vi "启动条件判断.vi"(7 "时间源":T1, 8 "仪器状态":bool, 9 "启动次数":i32, 10 "间隔计时":i32, 11 "周期设置输出":T6 {"定点周期"."启动命令 24" items=["", "水样测试", "标样核查", "零点核查", "跨度核查", "空白测试", "平行样测试", "加标回收", "空白校准", "标样校准"]; "定点周期"."启动命令 23" items=["", "水样测试", "标样核查", "零点核查", "跨度核查", "空白测试", "平行样测试", "加标回收", "空白校准", "标样校准"]; "定点周期"."启动命令 22" items=["", "水样测试", "标样核查", "零点核查", "跨度核查", "空白测试", "平行样测试", "加标回收", "空白校准", "标样校准"]; "定点周期"."启动命令 21" items=["", "水样测试", "标样核查", "零点核查", "跨度核查", "空白测试", "平行样测试", "加标回收", "空白校准", "标样校准"]; "定点周期"."启动命令 20" items=["", "水样测试", "标样核查", "零点核查", "跨度核查", "空白测试", "平行样测试", "加标回收", "空白校准", "标样校准"]; "定点周期"."启动命令 19" items=["", "水样测试", "标样核查", "零点核查", "跨度核查", "空白测试", "平行样测试", "加标回收", "空白校准", "标样校准"]; "定点周期"."启动命令 18" items=["", "水样测试", "标样核查", "零点核查", "跨度核查", "空白测试", "平行样测试", "加标回收", "空白校准", "标样校准"]; "定点周期"."启动命令 17" items=["", "水样测试", "标样核查", "零点核查", "跨度核查", "空白测试", "平行样测试", "加标回收", "空白校准", "标样校准"]; "定点周期"."启动命令 16" items=["", "水样测试", "标样核查", "零点核查", "跨度核查", "空白测试", "平行样测试", "加标回收", "空白校准", "标样校准"]; "定点周期"."启动命令 15" items=["", "水样测试", "标样核查", "零点核查", "跨度核查", "空白测试", "平行样测试", "加标回收", "空白校准", "标样校准"]; "定点周期"."启动命令 14" items=["", "水样测试", "标样核查", "零点核查", "跨度核查", "空白测试", "平行样测试", "加标回收", "空白校准", "标样校准"]; "定点周期"."启动命令 13" items=["", "水样测试", "标样核查", "零点核查", "跨度核查", "空白测试", "平行样测试", "加标回收", "空白校准", "标样校准"]; "定点周期"."启动命令 12" items=["", "水样测试", "标样核查", "零点核查", "跨度核查", "空白测试", "平行样测试", "加标回收", "空白校准", "标样校准"]; "定点周期"."启动命令 11" items=["", "水样测试", "标样核查", "零点核查", "跨度核查", "空白测试", "平行样测试", "加标回收", "空白校准", "标样校准"]; "定点周期"."启动命令 10" items=["", "水样测试", "标样核查", "零点核查", "跨度核查", "空白测试", "平行样测试", "加标回收", "空白校准", "标样校准"]; "定点周期"."启动命令 9" items=["", "水样测试", "标样核查", "零点核查", "跨度核查", "空白测试", "平行样测试", "加标回收", "空白校准", "标样校准"]; "定点周期"."启动命令 8" items=["", "水样测试", "标样核查", "零点核查", "跨度核查", "空白测试", "平行样测试", "加标回收", "空白校准", "标样校准"]; "定点周期"."启动命令 7" items=["", "水样测试", "标样核查", "零点核查", "跨度核查", "空白测试", "平行样测试", "加标回收", "空白校准", "标样校准"]; "定点周期"."启动命令 6" items=["", "水样测试", "标样核查", "零点核查", "跨度核查", "空白测试", "平行样测试", "加标回收", "空白校准", "标样校准"]; "定点周期"."启动命令 5" items=["", "水样测试", "标样核查", "零点核查", "跨度核查", "空白测试", "平行样测试", "加标回收", "空白校准", "标样校准"]; "定点周期"."启动命令 4" items=["", "水样测试", "标样核查", "零点核查", "跨度核查", "空白测试", "平行样测试", "加标回收", "空白校准", "标样校准"]; "定点周期"."启动命令 3" items=["", "水样测试", "标样核查", "零点核查", "跨度核查", "空白测试", "平行样测试", "加标回收", "空白校准", "标样校准"]; "定点周期"."启动命令 2" items=["", "水样测试", "标样核查", "零点核查", "跨度核查", "空白测试", "平行样测试", "加标回收", "空白校准", "标样校准"]; "定点周期"."启动命令" items=["", "水样测试", "标样核查", "零点核查", "跨度核查", "空白测试", "平行样测试", "加标回收", "空白校准", "标样校准"]; "间隔设置"."启动命令" items=["", "水样测试", "标样核查", "零点核查", "跨度核查", "空白测试", "平行样测试", "加标回收", "空白校准", "标样校准"]}) -> (2 "重新配置":bool, 3 "Data":T7 caption="数据")   [LabVIEW 2016, in "定时设置.xctl"]
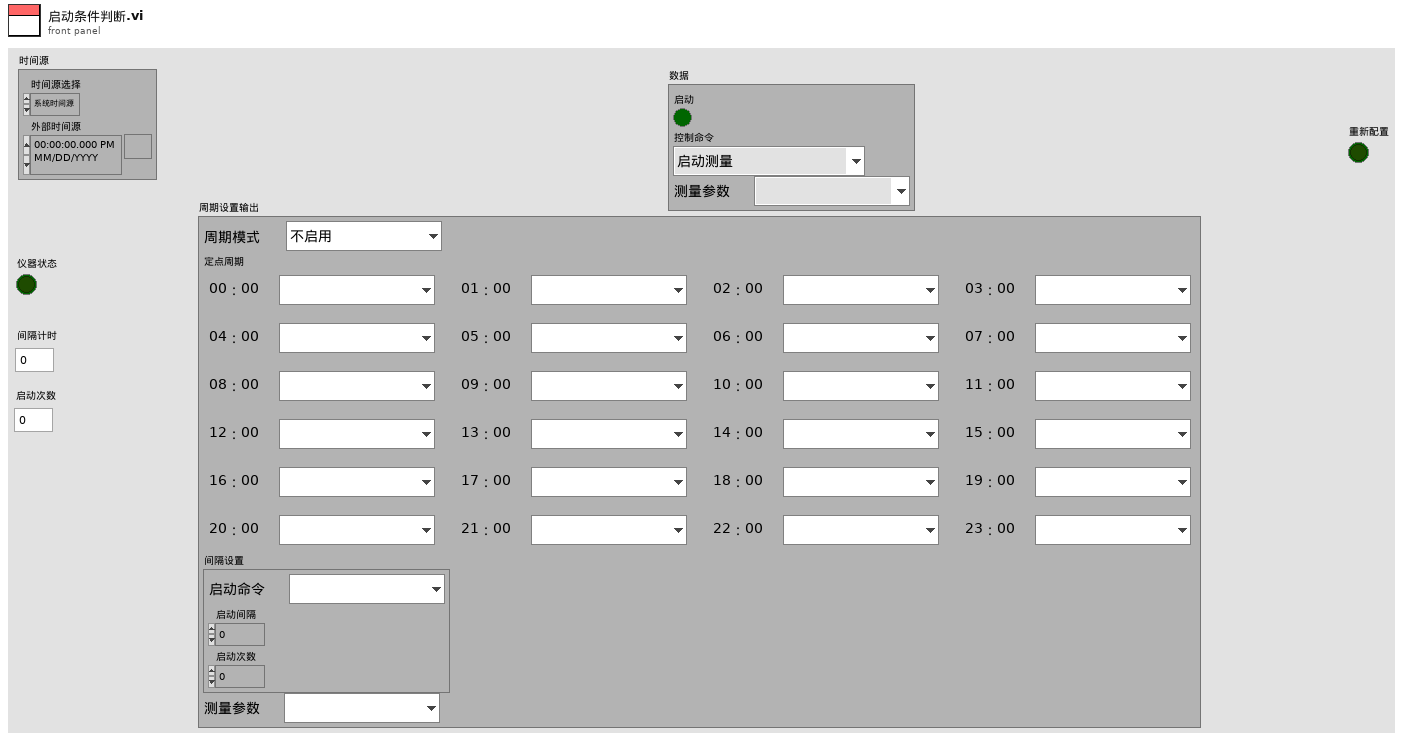
[diagram p1: front panel]
types:
  T1 = cluster{"时间源选择":enum16{"系统时间源", "仪器时间源"}, "外部时间源":timestamp}
  T2 = typedef "定时设置.xctl/周期模式设置.ctl" = enum16{"不启用", "定点模式", "间隔模式"}
  T3 = typedef "定时设置.xctl/定点周期设置.ctl" = cluster{"启动命令":T4, "启动命令 2":T4, "启动命令 3":T4, "启动命令 4":T4, "启动命令 5":T4, "启动命令 6":T4, "启动命令 7":T4, "启动命令 8":T4, "启动命令 9":T4, "启动命令 10":T4, "启动命令 11":T4, "启动命令 12":T4, "启动命令 13":T4, "启动命令 14":T4, "启动命令 15":T4, "启动命令 16":T4, "启动命令 17":T4, "启动命令 18":T4, "启动命令 19":T4, "启动命令 20":T4, "启动命令 21":T4, "启动命令 22":T4, "启动命令 23":T4, "启动命令 24":T4}
  T4 = typedef "定时设置.xctl/启动命令选择.ctl" = u16
  T5 = typedef "定时设置.xctl/测量参数.ctl" = u16
  T6 = cluster{"周期模式":T2, "定点周期":T3, "间隔设置":cluster{"启动命令":T4, "启动间隔":dbl, "启动次数":i32}, "测量参数":T5}
  T7 = typedef "定时设置.xctl/数据.ctl" = cluster{"启动":bool, "控制命令":T8, "测量参数":T5}
  T8 = typedef "定时设置.xctl/国标控制命令.ctl" = enum16{"启动测量", "标样核查", "零点核查", "跨度核查", "空白测试", "平行样测试", "加标回收", "空白校准", "标样校准", "初始化（清洗）", "停止测试", "仪器重启", "校时", "模式设置", "测量间隔设置"}
  T9 = typedef "LVDateTimeRec.ctl" = cluster{"秒数的小数部分":dbl, "秒":i32, "分":i32, "时":i32, "日":i32, "月":i32, "年":i32, "天数（周）":i32, "天数（年）":i32, "DST":i32}
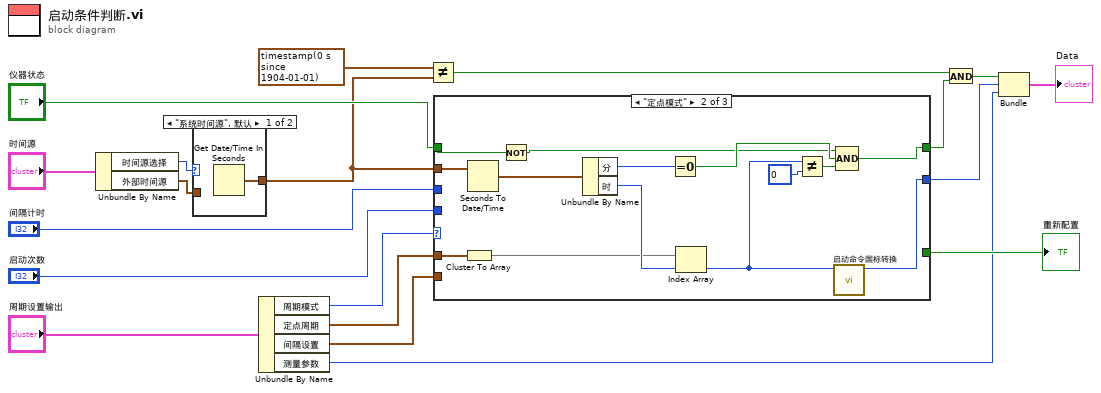
[diagram p0: block diagram]
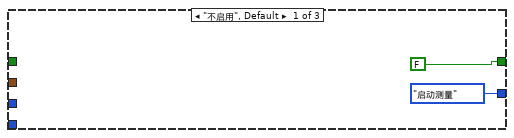
[diagram p3: hidden frame]
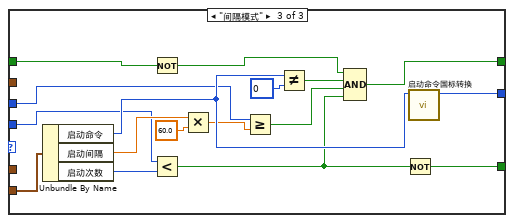
[diagram p4: hidden frame]
diagram:
  n1 = Unbundle By Name("时间源") -> ("时间源选择"=w6:enum16{"系统时间源", "仪器时间源"}, "外部时间源"=w5:timestamp)
  n2 = case shown="\"系统时间源\", 默认" w6 {
    tunnel: [w20 w21] -> w4
    tunnel: w5 -> [_ w21]
    frame "系统时间源", Default {
      n3 = Get Date/Time In Seconds() -> (seconds since 1Jan1904=w20:timestamp)
    }
    frame "仪器时间源" {
    }
  }
  n4 = Unbundle By Name("周期设置输出") -> ("周期模式"=w19:T2, "定点周期"=w18:T3, "间隔设置"=w17:cluster{"启动命令":T4, "启动间隔":dbl, "启动次数":i32}, "测量参数"=w8:T5)
  n5 = Not Equal?(x=timestamp(0 s since 1904-01-01), y=w4) -> (x != y?=w1:bool)
  n6 = case shown="\"定点模式\"" w19 {
    tunnel: w18 -> [_ w28 _]
    tunnel: w17 -> [_ _ w54]
    tunnel: [国标控制命令."启动测量" ("控制命令") w30 w53] -> w15
    tunnel: [FALSE w29 w44] -> w10
    tunnel: "启动次数" -> [_ _ w48]
    tunnel: "间隔计时" -> [_ _ w42]
    tunnel: "仪器状态" -> [_ w25 w41]
    tunnel: [_ _ w38] -> w9
    tunnel: w4 -> [_ w26 _]
    frame "不启用", Default {
    }
    frame "定点模式" {
      w35 = T4 0 items=["", "水样测试", "标样核查", "零点核查", "跨度核查", "空白测试", "平行样测试", "加标回收", "空白校准", "标样校准"] ("y")
      n7 = Cluster To Array(cluster=w28) -> (array=w27:T4[])
      n8 = Seconds To Date/Time(time stamp (now)=w26) -> (date time rec=w37:T9)  [unwired: 1 in]
      n9 = Not(x=w25) -> (.not. x?=w24:bool)
      n10 = Unbundle By Name(w37) -> ("分"=w34:i32, "时"=w36:i32)
      n11 = Equal To 0?(x=w34) -> (x = 0?=w32:bool)
      n12 = Index Array(array=w27, index=w36) -> (element=w31:T4)
      n13 = Not Equal?(x=w31, y=w35) -> (x != y?=w33:bool)
      n14 = call "启动命令国标转换.vi"("启动命令"=w31) -> ("控制命令"=w30:T8)  [unwired: 10 in]
      n15 = Compound Arithmetic op=AND ("复合运算")(w24, w32, w33) -> (w29:bool)
    }
    frame "间隔模式" {
      w51 = T4 0 items=["", "水样测试", "标样核查", "零点核查", "跨度核查", "空白测试", "平行样测试", "加标回收", "空白校准", "标样校准"] ("y")
      n16 = Unbundle By Name(w54) -> ("启动命令"=w52:T4, "启动间隔"=w50:dbl, "启动次数"=w47:i32)
      n17 = Not(x=w41) -> (.not. x?=w40:bool)
      n18 = Less?(x=w48, y=w47) -> (x < y?=w39:bool)
      n19 = Multiply(x=w50, y=60.0) -> (x*y=w43:dbl)
      n20 = Greater Or Equal?(x=w42, y=w43) -> (x >= y?=w45:bool)
      n21 = Not Equal?(x=w52, y=w51) -> (x != y?=w46:bool)
      n22 = Compound Arithmetic op=AND ("复合运算")(w40, w46, w45, w39) -> (w44:bool)
      n23 = Not(x=w39) -> (.not. x?=w38:bool)
      n24 = call "启动命令国标转换.vi"("启动命令"=w52) -> ("控制命令"=w53:T8)  [unwired: 10 in]
    }
  }
  "重新配置" <- w9
  n25 = And(x=w1, y=w10) -> (x .and. y?=w2:bool)
  n26 = Bundle(w2, "控制命令"=w15, "测量参数"=w8) -> (→"Data":cluster{bool, "控制命令":T8, "测量参数":T5})  [unwired: 1 in]
